vi "DSF.Execution.Builder.Get Plugin Buffer.vi"(8 "error in (no error)":errorcluster, 9 "timeout ms (0)":i32 format="%d ms", 10 "plugin id":i32, 11 "Builder in":refnum<class "DSF.Execution.Builder.lvclass">) -> (0 "error out":errorcluster, 1 "timed out?":bool, 2 "Buffer":refnum<class "DSF.Memory.Buffer.lvclass">, 3 "Builder out":refnum<class "DSF.Execution.Builder.lvclass">)   [LabVIEW 2016, in "DSF.Engine.lvlib" / "DSF.Execution.Builder.lvclass"]
uses:
  DSF.Execution.Builder.lvclass
  Memory.Buffer/DSF.Memory.Buffer.lvclass
  DSF.Execution.Builder.lvclass/DSF.Execution.Builder.ctl
  Memory.BufferPool/DSF.Memory.BufferPool.lvclass/DSF.Memory.BufferPool.ctl
  DSF.Execution.Builder.Get Plugin Buffer Pools.vi
  Memory.BufferPool/DSF.Memory.BufferPool.Get Index FIFO.vi
  Memory.BufferPool/DSF.Memory.BufferPool.Get Buffers.vi
  Memory.BufferPool/DSF.Memory.BufferPool.lvclass
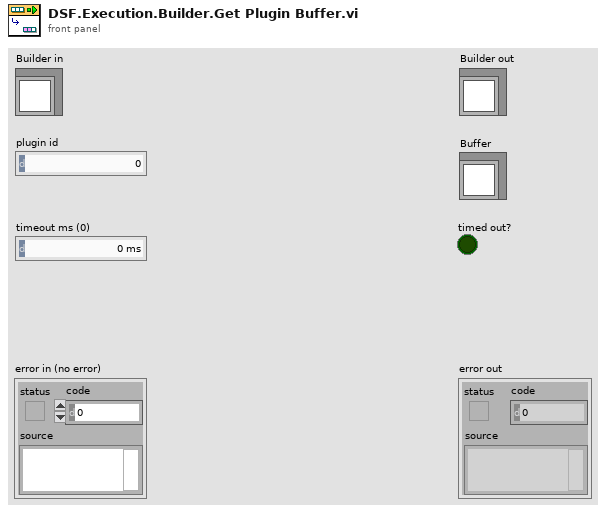
[diagram p1: front panel]
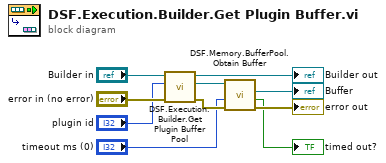
[diagram p0: block diagram]
diagram:
  n1 = call "DSF.Execution.Builder.Get Plugin Buffer Pool.vi"("error in (no error)"="error in (no error)", "plugin id"="plugin id", "Builder in"="Builder in") -> ("error out"=w6:errorcluster, "BufferPool"=w7:refnum<class "DSF.Memory.BufferPool.lvclass">, "Builder out"=→"Builder out":refnum<class "DSF.Execution.Builder.lvclass">)  [unwired: 6 in]
  n2 = call "DSF.Memory.BufferPool.Obtain Buffer.vi"("error in (no error)"=w6, "timeout ms (0)"="timeout ms (0)", "BufferPool in"=w7) -> ("error out"=→"error out":errorcluster, "timed out?"=→"timed out?":bool, "Buffer"=→"Buffer":refnum<class "DSF.Memory.Buffer.lvclass">)  [unwired: 5 in, 1 out]
